vi "Module Init.vi"(8 "error in (no error)":errorcluster, 11 "Git Updater Module in":refnum<class "Git Updater Module.lvclass">) -> (0 "error out":errorcluster, 3 "Git Updater Module out":refnum<class "Git Updater Module.lvclass">)   [LabVIEW 2020, in "VolatusGUI.lvlib" / "Git Updater Module.lvclass"]
uses:
  Git Updater Module.lvclass
  C:/dev/lv20CE/relink/lv-volatus/Volatus/Module/Module.lvclass
  Volatus/Module/Module.lvclass/Module.ctl
  Volatus/MessageQ/MessageQ.lvclass/MessageQ.ctl
  Volatus/Module/Self Q.vi
  Volatus/MessageQ/Send.vi
  Volatus/Module/Module.lvclass
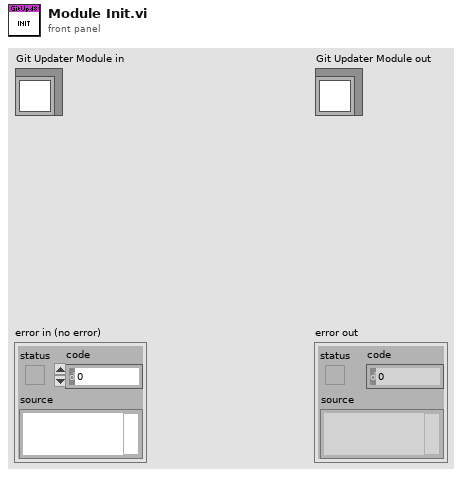
[diagram p1: front panel]
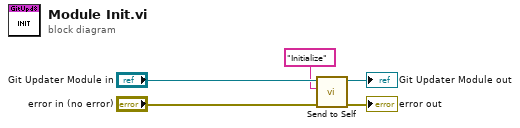
[diagram p0: block diagram]
diagram:
  n1 = call "Send to Self.vi"("error in (no error)"="error in (no error)", "Message ID"="Initialize", "Module in"="Git Updater Module in") -> ("error out"=→"error out":errorcluster, "Module out"=→"Git Updater Module out":refnum<class "Git Updater Module.lvclass">)  [unwired: 7 in]
